vi "Global_flags.vi"() -> ()   [LabVIEW 2021]
panel:
  in  "Calib Data?":bool
  in  "Adquire /Stop DATA?":bool
  in  "Open / Close COM?":bool
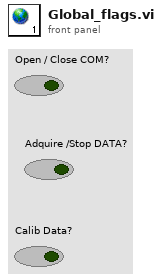
[diagram p1: front panel]
diagram:
